vi "WPI_CounterCache.vi"(8 "error in (no error)":errorcluster, 9 "CntIndexToRelease":T1=enum."Ctr 1", 11 "Operation":T2) -> (0 "error out":errorcluster, 2 "CntIndexAllocated":T1=enum."Ctr 1", 3 "Allocated":bool)   [LabVIEW 2017]
doc: "This software is licensed. Open the labview\\readme\\WPI Robotics Library Open Source License.txt file for more information."
uses:
  <vilib>/Rock Robotics/WPI/Counter/WPI_CounterCacheOp.ctl
  <vilib>/Rock Robotics/SystemInterfaces/Counter/FPGA_CounterCtrSystemIndex.ctl
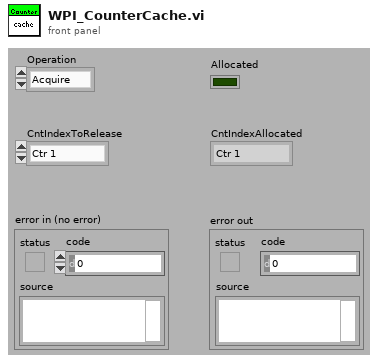
[diagram p1: front panel]
types:
  T1 = typedef "FPGA_CounterCtrSystemIndex.ctl" = enum8{"Ctr 0", "Ctr 1", "Ctr 2", "Ctr 3", "Ctr 4", "Ctr 5", "Ctr 6", "Ctr 7", "Invalid"}
  T2 = typedef "WPI_CounterCacheOp.ctl" = enum16{"Acquire", "Release"}
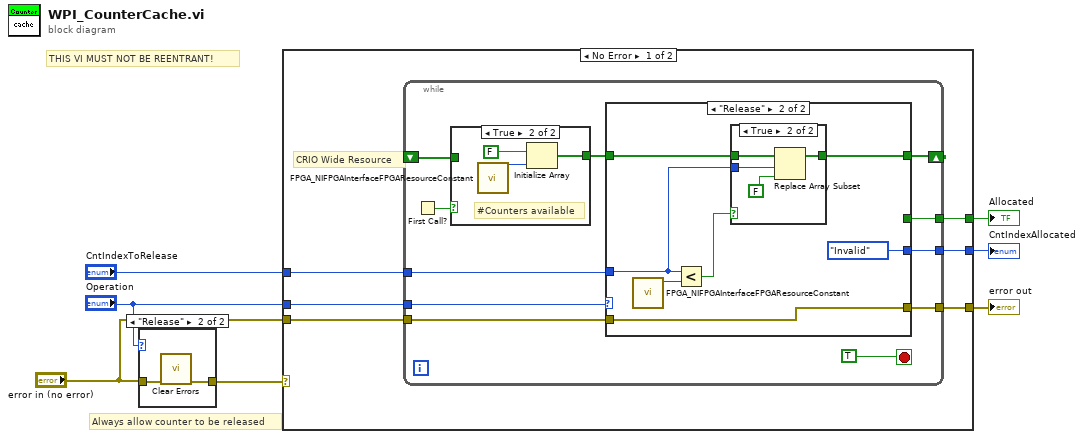
[diagram p0: block diagram]
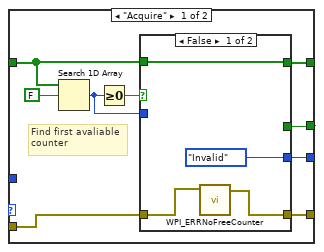
[diagram p3: hidden frame]
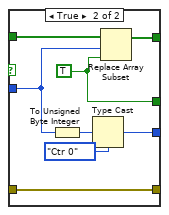
[diagram p4: hidden frame]
diagram:
  # "THIS VI MUST NOT BE REENTRANT!"
  # "Always allow counter to be released"
  n1 = case shown="\"Release\"" "Operation" {
    tunnel: "error in (no error)" -> [w8 w10]
    tunnel: [w8 w9] -> w5
    frame "Acquire", Default {
    }
    frame "Release" {
      n2 = call <vilib>:"Clear Errors.vi"("error in (no error)"=w10) -> ("error out"=w9:errorcluster)  [unwired: 1 in, 5 out]
    }
  }
  n3 = case shown="No Error" w5 {
    selector: w5 -> [_ w65]
    tunnel: "Operation" -> [w16 _]
    tunnel: [w15 w65] -> w1
    tunnel: [w14 _] -> w7
    tunnel: "CntIndexToRelease" -> [w12 _]
    tunnel: [w13 _] -> w3
    tunnel: "error in (no error)" -> [w11 _]
    frame No Error {
      # "CRIO Wide Resource"
      n4 = while {
        shift-right: [w24] -> _
        shift-left: _ -> [w26]
        tunnel: w16 -> [w25]
        tunnel: w12 -> [w20]
        tunnel: [w23] -> w15
        tunnel: [w22] -> w14
        tunnel: [w19] -> w13
        tunnel: w11 -> [w17]
        stop <- TRUE stop-if-true
        n5 = First Call?() -> (First Call?: T/F=w27:bool)
        n6 = case shown="True" w27 {
          tunnel: w26 -> [w61 _]
          tunnel: [w61 w63] -> w21
          frame False {
          }
          frame True {
            # "#Counters available"
            n7 = call <vilib>:"FPGA_NIFPGAInterfaceFPGAResourceConstant.vi"() -> ("NumberOfCounters"=w62:u32)  [unwired: 11 out]
            n8 = Initialize Array(FALSE, w62) -> (w63:bool[])
          }
        }
        n9 = case shown="\"Release\"" w25 {
          tunnel: w21 -> [w32 w55]
          tunnel: [w36 w54] -> w24
          tunnel: w20 -> [_ w51]
          tunnel: [w35 w52] -> w23
          tunnel: [w34 _] -> w22
          tunnel: [w33 FPGA_CounterCtrSystemIndex."Invalid" ("CntIndexToRelease")] -> w19
          tunnel: w17 -> [w28 w52]
          frame "Acquire" {
            # "Find first avaliable\ncounter"
            n10 = Search 1D Array(1D array=w32, element=FALSE) -> (index of element=w29:i32)  [unwired: 1 out]
            n11 = Greater Or Equal To 0?(x=w29) -> (x >= 0?=w30:bool)
            n12 = case shown="False" w30 {
              tunnel: w32 -> [w40 w47]
              tunnel: [w40 w46] -> w36
              tunnel: w29 -> [_ w44]
              tunnel: [w38 w41] -> w35
              tunnel: [_ w48] -> w34
              tunnel: [FPGA_CounterCtrSystemIndex."Invalid" ("CntIndexToRelease") w43] -> w33
              tunnel: w28 -> [w37 w41]
              frame False {
                n13 = call <vilib>:"WPI_ERRNoFreeCounter.vi"("error in (no error)"=w37) -> ("CounterAllocation"=w38:errorcluster)  [unwired: 10 out]
              }
              frame True {
                w48 = TRUE ("new element/subarray")
                n14 = To Unsigned Byte Integer(number=w44) -> (unsigned 8bit integer=w42:u8)
                n15 = Type Cast(type=FPGA_CounterCtrSystemIndex."Ctr 0" ("CntIndexToRelease"), x=w42) -> (*(type *) &x=w43:T1)
                n16 = Replace Array Subset(array=w47, new element=w48, index=w44) -> (w46:bool[])
              }
            }
          }
          frame "Release" {
            n17 = call <vilib>:"FPGA_NIFPGAInterfaceFPGAResourceConstant.vi"() -> ("NumberOfCounters"=w49:u32)  [unwired: 11 out]
            n18 = Less?(x=w51, y=w49) -> (x < y?=w50:bool)
            n19 = case shown="True" w50 {
              tunnel: w55 -> [w56 w60]
              tunnel: [w56 w59] -> w54
              tunnel: w51 -> [_ w58]
              frame False {
              }
              frame True {
                n20 = Replace Array Subset(array=w60, new element=FALSE ("new element/subarray"), index=w58) -> (w59:bool[])
              }
            }
          }
        }
      }
    }
    frame Error {
    }
  }
  "Allocated" <- w7
  "error out" <- w1
  "CntIndexAllocated" <- w3
